vi "Configure Current Limit.vi"(0 "reference in":refnum<class "BKP-911x Power Supply.lvclass">, 2 "Current Limit (0.0 A)":dbl format="%.3g", 5 "error in (no error)":errorcluster) -> (14 "reference out":refnum<class "BKP-911x Power Supply.lvclass">, 19 "error out":errorcluster)   [LabVIEW 2018, in "BKP-911x Power Supply.lvclass"]
uses:
  BKP-911x Power Supply.lvclass
  <instrlib>/BK Precision 911X Series/BK Precision 911X Series.lvlib
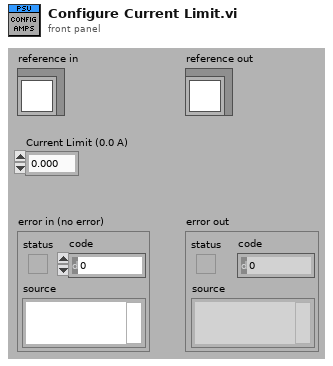
[diagram p1: front panel]
types:
  T1 = typedef "BKP-911x Power Supply.lvclass/ObjectAttributes.ctl" = cluster{"VISA resource name":refnum<visa-resource-name>, "Simulated?":bool, "Latest Values":dbl[], "Signal List":T2[], "Voltage Setpoint (V)":dbl, "Current Limit (A)":dbl, "Output Enabled?":bool}
  T2 = typedef "IO Signal List.ctl" = enum16{"Timestamp", "PSU_FB_U_VDC", "PSU_FB_I_AMP", "PSU_FB_W_WATT", "PSU_CMD_U_VDC", "PSU_CMD_I_AMP", "PSU_CMD_OUTPUT", "U_U_VDC", "V_U_VDC", "W_U_VDC", "U_I_AMP", "V_I_AMP", "W_I_AMP", "LCR_PRIMARY", "LCR_SECONDARY", "UV_R_mOhm", "UW_R_mOhm", "VW_R_mOhm", "UV_L_µH", "UW_L_µH", "VW_L_µH", "DIFF_UV_UW_L_µH", "DIFF_UV_VW_L_µH", "DIFF_UW_VW_L_µH", "DIFF_UV_UW_R_mOhm", "DIFF_UV_VW_R_mOhm", "DIFF_UW_VW_R_mOhm", "DIFF_UV_U_VDC", "DIFF_UW_U_VDC", "DIFF_VW_U_VDC", "PWM_CMD_DC_%", "PWM_CMD_VDC", "PWM_CMD_Hz", "PWM_FB_DC_%", "PWM_FB_VDC", "PWM_FB_Hz", "DO_RELAY_U_LCR_A", "DO_RELAY_V_LCR_A", "DO_RELAY_V_LCR_B", "DO_RELAY_W_LCR_B"}
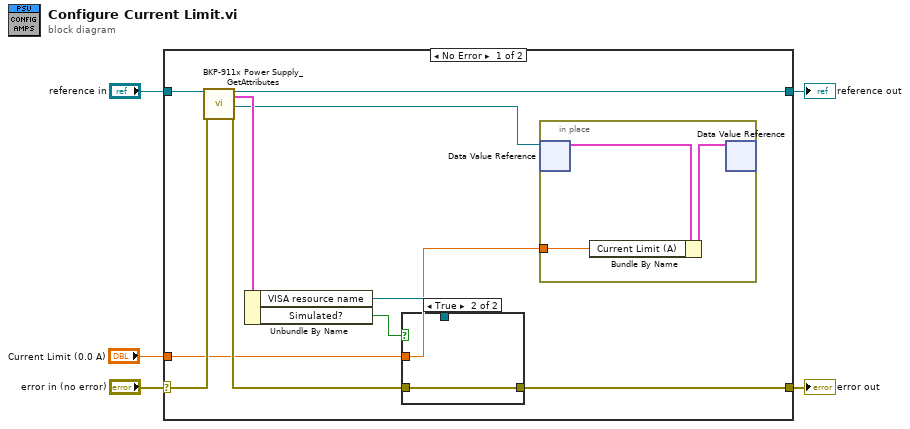
[diagram p0: block diagram]
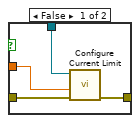
[diagram p2: hidden frame]
diagram:
  n1 = case shown="No Error" "error in (no error)" {
    selector: "error in (no error)" -> [w15 w25]
    tunnel: [w10 w25] -> w4
    tunnel: [w12 w24] -> w2
    tunnel: "reference in" -> [w13 w24]
    tunnel: "Current Limit (0.0 A)" -> [w7 _]
    frame No Error {
      n2 = call "BKP-911x Power Supply_GetAttributes.vi"("reference in"=w13, "error in (no error)"=w15) -> ("reference out"=w12:refnum<class "BKP-911x Power Supply.lvclass">, "Data"=w14:T1, "DataRef"=w8:refnum<data-value>, "error out"=w11:errorcluster)  [unwired: 14 in]
      n3 = Unbundle By Name(w14) -> ("VISA resource name"=w9:refnum<visa-resource-name>, "Simulated?"=w6:bool)
      n4 = case shown="True" w6 {
        tunnel: w11 -> [w19 w20]
        tunnel: [w18 w20] -> w10
        tunnel: w9 -> [w17 _]
        tunnel: w7 -> [w16 _]
        frame False {
          n5 = call <instrlib>:"Configure Current Limit.vi"("error in (no error)"=w19, "Current Limit (0.0 A)"=w16, "VISA resource name"=w17) -> ("error out"=w18:errorcluster)  [unwired: 7 in, 1 out]
        }
        frame True {
        }
      }
      n6 = in-place {
        in-place-border: w7 -> [w21]
        n7 = in-place-dvr #1(w8) -> (w23:T1)  [unwired: 1 out]
        n8 = Bundle By Name(cluster=w23, "Current Limit (A)"=w21) -> (w22:T1)
        n9 = in-place-dvr #1(w22) -> ()  [unwired: 2 out]
      }
    }
    frame Error {
    }
  }
  "error out" <- w4
  "reference out" <- w2
